vi "SMO.TimedLoop.DVRtoRef.vi"(10 "Ref":T1) -> (2 "Ref":u32 format="%08x")   [LabVIEW 2013, in "SMO.TimedLoop.lvclass"]
doc: "JKI State Machine Objects (SMO) 1.0.0.5\nJKI - JKI\nCopyright (c) 2016, JKI"
uses:
  SMO.TimedLoop.lvclass
  Typedefs/PrivateData--Ref.ctl
  Typedefs/PrivateData--Cluster.ctl
  Typedefs/PublicEvents--Cluster.ctl
  Typedefs/SetpointChanged--EventData--Cluster.ctl
  Typedefs/Data.ctl
  Typedefs/PrivateEvents--Cluster.ctl
  Typedefs/AsyncMethodInputs--Cluster.ctl
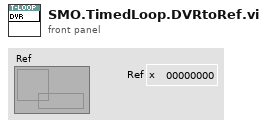
[diagram p1: front panel]
types:
  T1 = typedef "SMO.TimedLoop.lvclass/PrivateData--Ref.ctl" = refnum<data-value>
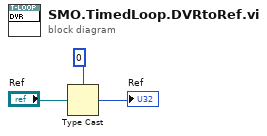
[diagram p0: block diagram]
diagram:
  n1 = Type Cast(type=u32 0 ("Ref"), x="Ref") -> (*(type *) &x=→"Ref":u32)
